vi "Front Panel Globals.vi"() -> ()   [LabVIEW 2023]
uses:
  <vilib>/LabVIEW Targets/FPGA/cRIO/shared/nicrio_ModuleControls/nicrio_cRIO-9467_Altitude.ctl
  <vilib>/LabVIEW Targets/FPGA/cRIO/shared/nicrio_ModuleControls/nicrio_cRIO-9467_Longitude.ctl
  <vilib>/LabVIEW Targets/FPGA/cRIO/shared/nicrio_ModuleControls/nicrio_cRIO-9467_Latitude.ctl
panel:
  out "Analog Data Down":sgl[](array[numeric])
  in  "PPS Count Ticks":u32
  out "PPS Trigger Count":u32
  out "PPS Trigger":bool
  out "PPS Counter Loops":i32
  out "FPGA Analog Data Length":i32
  out "Analog Data Up":sgl[](array[numeric])
  out "GPS Latitude (°)":T1 format="%.6f"
  out "GPS Longitude (°)":T2 format="%.6g"
  out "GPS Altitude (m)":T3 format="%.2f"
  out "GPS Self-Survey Complete":bool
  out "GPS Vendor ID":u16
  out "GPS Firmware Version":u32
  out "GPS Serial Number":u32
  out "Watchdog Whack Count":u32
  out "Watchdog ms Since Whack":u32
  in  "Watchdog Timeout (ms)":u32=3600000
  in  "FPGA System Reset":bool
  in  "FPGA USER1 LED":bool
  in  "Watchdog Whack":bool
  in  "Watchdog Enable":bool
  out "FPGA Nanosecond Counter":u64
  out "GPS Time Lock":bool
  out "GPS Time (ns)":u64
  out "GPS Status":T4(ring)
  out "GPS Time Offset":i32
  out "GPS Antenna Status":T5(ring)
  out "GPS Satelites Available":u8
  out "GPS UTC Offset":i8
  out "GPS UTC Offset Valid":bool
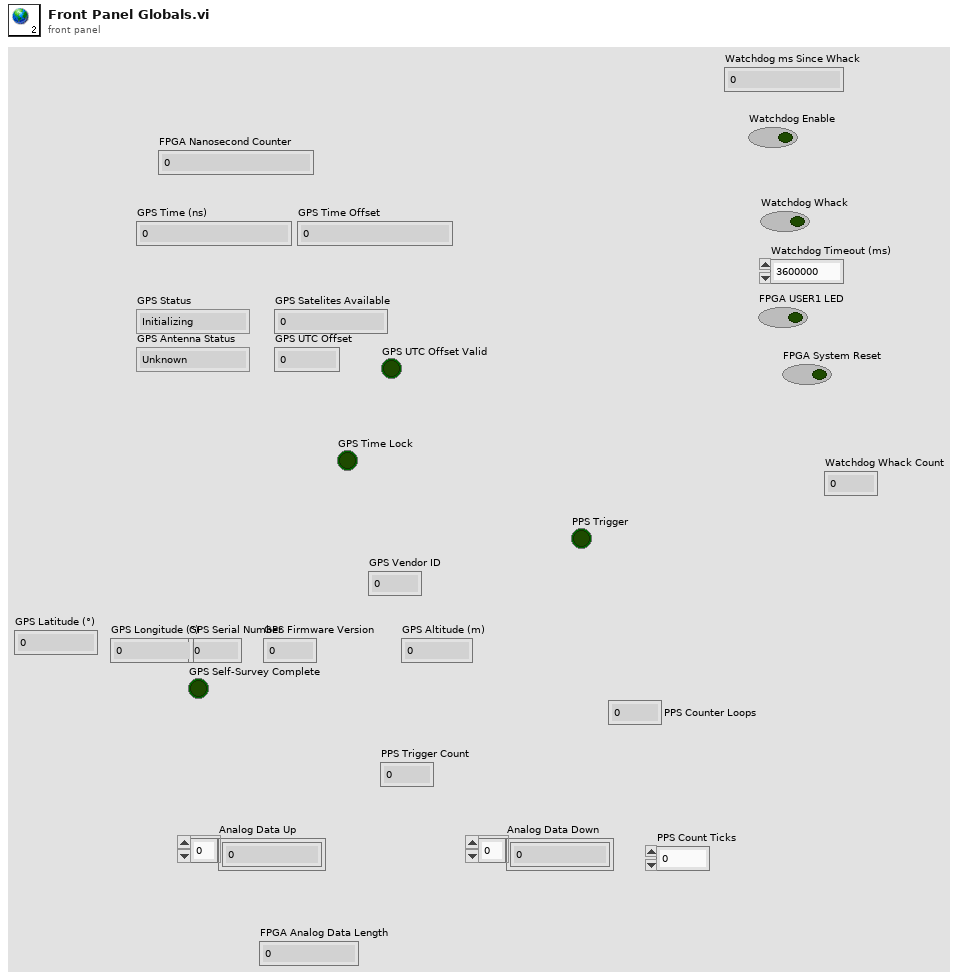
[diagram p1: front panel]
types:
  T1 = typedef "nicrio_cRIO-9467_Latitude.ctl" = fxp<+/-,28,8>
  T2 = typedef "nicrio_cRIO-9467_Longitude.ctl" = fxp<+/-,29,9>
  T3 = typedef "nicrio_cRIO-9467_Altitude.ctl" = fxp<+/-,24,17>
  T4 = enum8{"Initializing", "Normal", "Unable to get fix"}
  T5 = enum8{"Unknown", "Normal", "Absent", "Overcurrent"}
diagram:
